vi "TDMS to HDF5.vi"() -> ()   [LabVIEW 2012]
uses:
  TDMSdatatype.ctl
  <vilib>/addons/_hdf5/group.llb/OpenCreateGroup (String).vi
  TDMS chan to HDF5 (i16).vi
  TDMS chan to HDF5 (i32).vi
  TDMS chan to HDF5 (dbl).vi
  TDMS chan to HDF5 (str).vi
panel:
  out "totalsets":i16
  out "setnum":i16
  out "totalfiles":i32
  out "filenum":i32
  out "File progress":dbl(slide) scale=0.0..1.0
  out "Dataset":string
  out "Total progress":dbl(slide) scale=0.0..1.0
  out "Current file":string
  # "of"
  # "of"
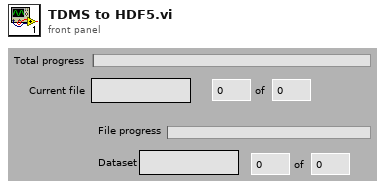
[diagram p1: front panel]
types:
  T1 = enum16{"open", "open or create", "create or replace", "create", "open (read-only)"}
  T2 = enum16{"open", "open or create", "create or replace", "create", "open (read only)"}
  T3 = typedef "HDF5 Ref.ctl" = refnum<k1>
  T4 = typedef "TDMSdatatype.ctl" = u16
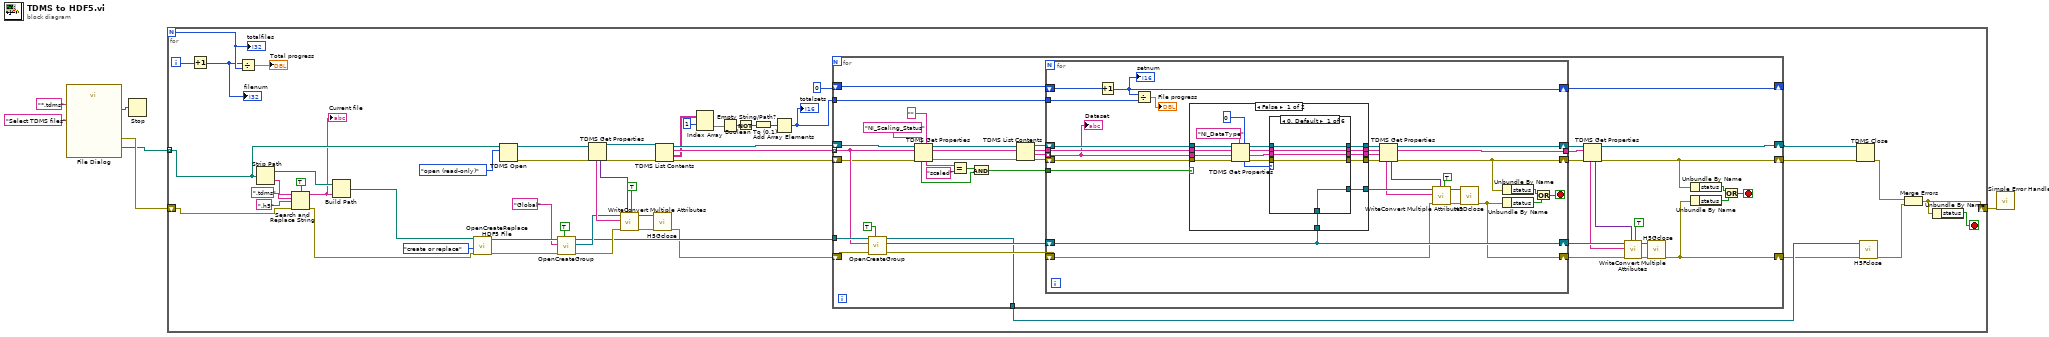
[diagram p0: block diagram]
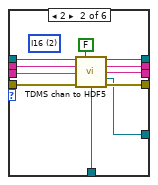
[diagram p2: hidden frame]
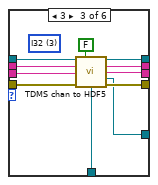
[diagram p3: hidden frame]
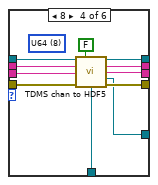
[diagram p4: hidden frame]
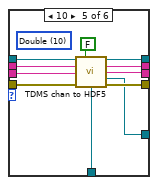
[diagram p5: hidden frame]
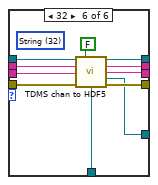
[diagram p6: hidden frame]
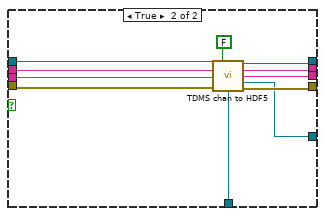
[diagram p7: hidden frame]
diagram:
  n1 = call "File Dialog"("prompt"="Select TDMS files", "pattern (all files)"="*.tdms") -> ("selected paths"=w1:path[], "cancelled"=w4:bool, "error out"=w2:errorcluster)  [unwired: 10 in, 1 out]
  n2 = Stop(stop? (T)=w4) -> ()
  n3 = for {
    N -> [w19]
    shift-right: [w9] -> w3
    shift-left: w2 -> [w23]
    tunnel: w1 -> [w27] mode=indexing
    i -> [w20]
    stop <- w8 stop-if-true
    n4 = Increment(x=w20) -> (x+1=w10:i32)
    "filenum" <- w10
    n5 = Divide(x=w10, y=w19) -> (x/y=→"Total progress":dbl)
    n6 = Strip Path(path=w27) -> (stripped path=w26:path, name=w31:string)
    n7 = Search and Replace String(case sensitive?=TRUE ("ignore case? (F)"), input string=w31, search string=".tdms", replace string=".h5" ("replace string (\"\")"), error in=w23) -> (result string=w25:string, error out=w22:errorcluster)  [unwired: 3 in, 2 out]
    "Current file" <- w25
    n8 = Build Path(base path=w26, name or relative path=w25) -> (appended path=w24:path)
    n9 = call <vilib>:"OpenCreateReplace HDF5 File.vi"("error in (no error)"=w22, "function (open:0)"=T2."create or replace", "path"=w24) -> ("error out"=w49:errorcluster, "HDF5 Ref out"=w51:T3)  [unwired: 5 in]
    n10 = TDMS Open(10:T1."open (read-only)" ("operation (0:open)"), 11:w27) -> (0:w44:errorcluster, 3:w45:refnum<k34>)  [unwired: 4 in]
    n11 = call-poly <vilib>:"OpenCreateGroup.vi"("Create if not found (F)"=TRUE, "error in (no error)"=w49, "Group"="Global", "HDF5 Ref"=w51) -> ("error out"=w40:errorcluster, "HDF5 Group Ref"=w41:T3, "HDF5 Ref out"=w39:T3)  [unwired: 3 in]
    n12 = TDMS Get Properties(8:w44, 11:w45) -> (0:w42:errorcluster, 3:w43:refnum<k34>, 4:w47:variant[], 6:w48:string[])  [unwired: 4 in, 2 out]
    n13 = call "WriteConvert Multiple Attributes.vi"("Replace Existing (F)"=TRUE, "Values"=w47, "error in (no error)"=w40, "Names"=w48, "HDF5 Ref"=w41) -> ("error out"=w37:errorcluster, "HDF5 Ref out"=w38:T3)  [unwired: 3 in]
    n14 = call <vilib>:"H5Gclose.vi"("error in (no error)"=w37, "HDF5 Group Ref"=w38) -> ("error out"=w36:errorcluster)  [unwired: 7 in]
    n15 = TDMS List Contents(4:w42, 7:w43) -> (0:w54:errorcluster, 1:w18:string[][], 2:w55:string[], 3:w56:refnum<k34>)  [unwired: 1 in]
    n16 = Index Array(array=w18, index (row)=1) -> (element=w16:string[])  [unwired: 1 in]
    n17 = Empty String/Path?(string/path=w16) -> (empty?=w15:bool[])
    n18 = Not(x=w15) -> (.not. x?=w14:bool[])
    n19 = Boolean To (0,1)(Boolean=w14) -> (0, 1=w13:i16[])
    n20 = Add Array Elements(numeric array=w13) -> (sum=w11:i16)
    "totalsets" <- w11
    n21 = for {
      tunnel: w55 -> [w73] mode=indexing
      tunnel: w39 -> [w100]
      shift-right: [w93] -> w33
      shift-left: w36 -> [w92]
      shift-right: [w87] -> w32
      shift-left: w54 -> [w71]
      tunnel: [w91] -> w34
      shift-right: [w61] -> _
      shift-left: i16 0 -> [w62]
      tunnel: w11 -> [w60]
      shift-right: [w59] -> w7
      shift-left: w56 -> [w72]
      stop <- w94 stop-if-true
      n22 = call-poly <vilib>:"OpenCreateGroup.vi"("Create if not found (F)"=TRUE, "error in (no error)"=w92, "Group"=w73, "HDF5 Ref"=w100) -> ("error out"=w97:errorcluster, "HDF5 Group Ref"=w98:T3, "HDF5 Ref out"=w91:T3)  [unwired: 3 in]
      n23 = TDMS Get Properties(5:"" ("property name"), 7:"NI_Scaling_Status" ("property name"), 8:w71, 10:w73, 11:w72) -> (0:w68:errorcluster, 2:w69:string, 3:w70:refnum<k34>, 4:w76:string, 6:w79:bool)  [unwired: 1 in, 1 out]
      n24 = Equal?(x=w76, y="scaled") -> (x = y?=w78:bool)
      n25 = And(x=w78, y=w79) -> (x .and. y?=w63:bool)
      n26 = TDMS List Contents(4:w68, 6:w69, 7:w70) -> (0:w64:errorcluster, 1:w65:string[], 2:w66:string, 3:w67:refnum<k34>)
      n27 = for {
        tunnel: w66 -> [w108]
        tunnel: w65 -> [w102] mode=indexing
        shift-right: [w113] -> w82
        shift-left: w97 -> [w120]
        shift-right: [w116] -> w88
        shift-left: w64 -> [w107]
        tunnel: [w110] -> w89
        tunnel: w63 -> [w106]
        shift-right: [w101] -> w61
        shift-left: w62 -> [w105]
        tunnel: w60 -> [w104]
        shift-right: [w111] -> w90
        shift-left: w67 -> [w109]
        shift-right: [w128] -> w86
        shift-left: w98 -> [w128]
        stop <- w112 stop-if-true
        n28 = Increment(x=w105) -> (x+1=w101:i16)
        "setnum" <- w101
        n29 = Divide(x=w101, y=w104) -> (x/y=→"File progress":dbl)
        n30 = case shown="False" w106 {
          tunnel: [w138 w210] -> w127
          tunnel: w128 -> [w137 w212]
          tunnel: [w136 w211] -> w126
          tunnel: w107 -> [w135 w213]
          tunnel: w102 -> [w134 w214]
          tunnel: w108 -> [w133 w215]
          tunnel: w109 -> [w132 w216]
          tunnel: [w131 w209] -> w125
          tunnel: [w130 w208] -> w124
          tunnel: [w129 w207] -> w123
          frame False {
            n31 = TDMS Get Properties(5:u16 0, 7:"NI_DataType" ("property name"), 8:w135, 9:w134, 10:w133, 11:w132) -> (0:w139:errorcluster, 1:w140:string, 2:w141:string, 3:w142:refnum<k34>, 4:w143:u16)  [unwired: 1 out]
            n32 = case shown="0, Default" w143 {
              tunnel: w142 -> [w149 w161 w172 w183 w194 w205]
              tunnel: w141 -> [w148 w160 w171 w182 w193 w204]
              tunnel: w140 -> [w147 w159 w170 w181 w192 w203]
              tunnel: w139 -> [w150 w158 w169 w180 w191 w202]
              tunnel: [w150 w157 w168 w179 w190 w201] -> w138
              tunnel: w137 -> [w146 w156 w167 w178 w189 w200]
              tunnel: [w149 w155 w166 w177 w188 w199] -> w136
              tunnel: [w148 w154 w165 w176 w187 w198] -> w131
              tunnel: [w147 w153 w164 w175 w186 w197] -> w130
              tunnel: [w146 w152 w163 w174 w184 w195] -> w129
              frame 0, Default {
              }
              frame 2 {
                (unwired) T4 2 items=["Void"=0, "I8"=1, "I16"=2, "I32"=3, "I64"=4, "U8"=5, "U16"=6, "U32"=7, "U64"=8, "Single"=9, "Double"=10, "Extended"=11, "SingleWUnit"=25, "DoubleWithUnit"=26, "ExtendedWithUnit"=27, "String"=32, "Boolean"=33, "TimeStamp"=68] ("TDMSdatatype")
                n33 = call-poly "TDMS chan to HDF5.vi"("tdms file"=w161, "close dataset? (T)"=FALSE, "group name in"=w160, "channel name in"=w159, "error in (no error)"=w158, "HDF5 Ref"=w156) -> ("tdms file out"=w155:refnum<k34>, "group name out"=w154:string, "channel name out"=w153:string, "dataset out"=w152:T3, "error out"=w157:errorcluster)  [unwired: 5 in]
              }
              frame 3 {
                (unwired) T4 3 items=["Void"=0, "I8"=1, "I16"=2, "I32"=3, "I64"=4, "U8"=5, "U16"=6, "U32"=7, "U64"=8, "Single"=9, "Double"=10, "Extended"=11, "SingleWUnit"=25, "DoubleWithUnit"=26, "ExtendedWithUnit"=27, "String"=32, "Boolean"=33, "TimeStamp"=68] ("TDMSdatatype")
                n34 = call-poly "TDMS chan to HDF5.vi"("tdms file"=w172, "close dataset? (T)"=FALSE, "group name in"=w171, "channel name in"=w170, "error in (no error)"=w169, "HDF5 Ref"=w167) -> ("tdms file out"=w166:refnum<k34>, "group name out"=w165:string, "channel name out"=w164:string, "dataset out"=w163:T3, "error out"=w168:errorcluster)  [unwired: 5 in]
              }
              frame 8 {
                (unwired) T4 8 items=["Void"=0, "I8"=1, "I16"=2, "I32"=3, "I64"=4, "U8"=5, "U16"=6, "U32"=7, "U64"=8, "Single"=9, "Double"=10, "Extended"=11, "SingleWUnit"=25, "DoubleWithUnit"=26, "ExtendedWithUnit"=27, "String"=32, "Boolean"=33, "TimeStamp"=68] ("TDMSdatatype")
                n35 = call-poly "TDMS chan to HDF5.vi"("tdms file"=w183, "close dataset? (T)"=FALSE, "group name in"=w182, "channel name in"=w181, "error in (no error)"=w180, "HDF5 Ref"=w178) -> ("tdms file out"=w177:refnum<k34>, "group name out"=w176:string, "channel name out"=w175:string, "dataset out"=w174:T3, "error out"=w179:errorcluster)  [unwired: 5 in]
              }
              frame 10 {
                (unwired) T4 10 items=["Void"=0, "I8"=1, "I16"=2, "I32"=3, "I64"=4, "U8"=5, "U16"=6, "U32"=7, "U64"=8, "Single"=9, "Double"=10, "Extended"=11, "SingleWUnit"=25, "DoubleWithUnit"=26, "ExtendedWithUnit"=27, "String"=32, "Boolean"=33, "TimeStamp"=68] ("TDMSdatatype")
                n36 = call-poly "TDMS chan to HDF5.vi"("tdms file"=w194, "close dataset? (T)"=FALSE, "group name in"=w193, "channel name in"=w192, "error in (no error)"=w191, "HDF5 Ref"=w189) -> ("tdms file out"=w188:refnum<k34>, "group name out"=w187:string, "channel name out"=w186:string, "dataset out"=w184:T3, "error out"=w190:errorcluster)  [unwired: 5 in]
              }
              frame 32 {
                (unwired) T4 32 items=["Void"=0, "I8"=1, "I16"=2, "I32"=3, "I64"=4, "U8"=5, "U16"=6, "U32"=7, "U64"=8, "Single"=9, "Double"=10, "Extended"=11, "SingleWUnit"=25, "DoubleWithUnit"=26, "ExtendedWithUnit"=27, "String"=32, "Boolean"=33, "TimeStamp"=68] ("TDMSdatatype")
                n37 = call-poly "TDMS chan to HDF5.vi"("tdms file"=w205, "close dataset? (T)"=FALSE, "group name in"=w204, "channel name in"=w203, "error in (no error)"=w202, "HDF5 Ref"=w200) -> ("tdms file out"=w199:refnum<k34>, "group name out"=w198:string, "channel name out"=w197:string, "dataset out"=w195:T3, "error out"=w201:errorcluster)  [unwired: 5 in]
              }
            }
          }
          frame True {
            n38 = call-poly "TDMS chan to HDF5.vi"("tdms file"=w216, "close dataset? (T)"=FALSE, "group name in"=w215, "channel name in"=w214, "error in (no error)"=w213, "HDF5 Ref"=w212) -> ("tdms file out"=w211:refnum<k34>, "group name out"=w209:string, "channel name out"=w208:string, "dataset out"=w207:T3, "error out"=w210:errorcluster)  [unwired: 5 in]
          }
        }
        n39 = TDMS Get Properties(8:w127, 9:w124, 10:w125, 11:w126) -> (0:w116:errorcluster, 2:w110:string, 3:w111:refnum<k34>, 4:w122:variant[], 6:w121:string[])  [unwired: 2 in, 1 out]
        n40 = call "WriteConvert Multiple Attributes.vi"("Replace Existing (F)"=TRUE, "Values"=w122, "error in (no error)"=w120, "Names"=w121, "HDF5 Ref"=w123) -> ("error out"=w115:errorcluster, "HDF5 Ref out"=w114:T3)  [unwired: 3 in]
        n41 = call <vilib>:"H5Dclose.vi"("error in (no error)"=w115, "HDF5 Dataset Ref"=w114) -> ("error out"=w113:errorcluster)  [unwired: 7 in]
        n42 = Unbundle By Name(w116) -> ("status"=w118:bool)
        n43 = Unbundle By Name(w113) -> ("status"=w117:bool)
        n44 = Or(x=w118, y=w117) -> (x .or. y?=w112:bool)
        "Dataset" <- w102
      }
      n45 = TDMS Get Properties(8:w88, 10:w89, 11:w90) -> (0:w87:errorcluster, 3:w59:refnum<k34>, 4:w84:variant[], 6:w85:string[])  [unwired: 3 in, 2 out]
      n46 = call "WriteConvert Multiple Attributes.vi"("Replace Existing (F)"=TRUE, "Values"=w84, "error in (no error)"=w82, "Names"=w85, "HDF5 Ref"=w86) -> ("error out"=w81:errorcluster, "HDF5 Ref out"=w80:T3)  [unwired: 3 in]
      n47 = call <vilib>:"H5Gclose.vi"("error in (no error)"=w81, "HDF5 Group Ref"=w80) -> ("error out"=w93:errorcluster)  [unwired: 7 in]
      n48 = Unbundle By Name(w87) -> ("status"=w95:bool)
      n49 = Unbundle By Name(w93) -> ("status"=w96:bool)
      n50 = Or(x=w95, y=w96) -> (x .or. y?=w94:bool)
    }
    n51 = TDMS Close(8:w32, 11:w7) -> (0:w53:errorcluster)  [unwired: 1 out]
    n52 = call <vilib>:"H5Fclose.vi"("error in (no error)"=w33, "HDF5 Ref"=w34) -> ("error out"=w52:errorcluster)  [unwired: 7 in]
    n53 = Merge Errors(w53, w52) -> (w9:errorcluster)
    n54 = Unbundle By Name(w9) -> ("status"=w8:bool)
    "totalfiles" <- w19
  }
  n55 = call <vilib>:"Simple Error Handler.vi"("error in (no error)"=w3) -> ()  [unwired: 4 in, 5 out]
